vi "Get Clicked Column Header.vi"(0 "TreeControl ref":refnum<vi>, 7 "Coords":T1, 11 "error in (no error)":errorcluster) -> (4 "TreeControl dup ref":refnum<vi>, 8 "Column #":i32, 15 "error out":errorcluster)   [LabVIEW 2015, in "QuickVIew.lvlib"]
doc: "TLB Prime - Application Template 1.3.0.24\nNorm Kirchner, NI Systems Engineering - NI\nCopyright (c) 2014, NI"
uses:
  QuickVIew.lvlib
  <vilib>/Utility/miscctls.llb/LVPoint32TypeDef.ctl
panel:
  # "VI LOCALS"
  # "VI OUTPUTS"
  # "VI INPUTS"
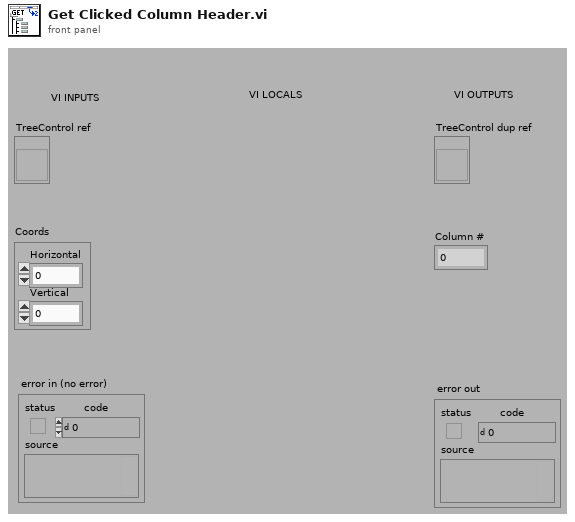
[diagram p1: front panel]
types:
  T1 = typedef "LVPoint32TypeDef.ctl" = cluster{"Horizontal":i32, "Vertical":i32}
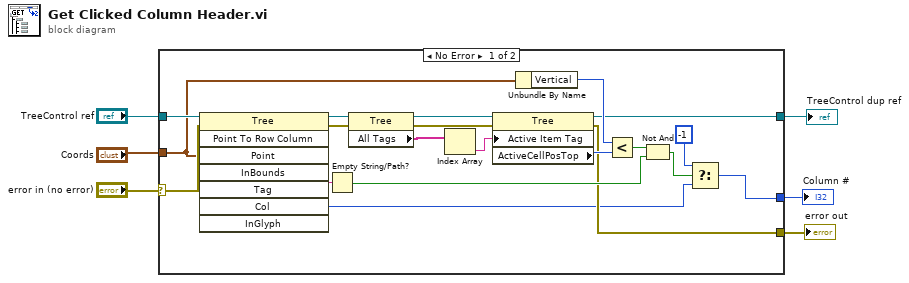
[diagram p0: block diagram]
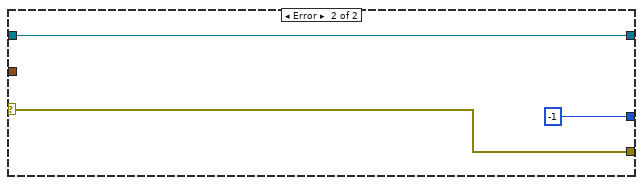
[diagram p2: hidden frame]
diagram:
  n1 = case shown="No Error" "error in (no error)" {
    selector: "error in (no error)" -> [w26 w27]
    tunnel: "TreeControl ref" -> [w25 w28]
    tunnel: "Coords" -> [w22 _]
    tunnel: [w7 -1 ("Col")] -> w4
    tunnel: [w12 w28] -> w2
    tunnel: [w9 w27] -> w1
    frame No Error {
      n2 = invoke on="Invoke Node" class="Tree" method="Point To Row Column"(reference=w25, error in=w26, "Point"=w22) -> (reference out=w23:refnum<vi>, error out=w11:errorcluster, "Tag"=w24:string, "Col"=w8:i32)  [unwired: 5 in, 4 out]
      n3 = Empty String/Path?(string/path=w24) -> (empty?=w15:bool)
      n4 = property class="Tree"(reference=w23, error in=w11) -> (reference out=w21:refnum<vi>, error out=w10:errorcluster, "All Tags"=w20:string[])
      n5 = Index Array(array=w20) -> (element=w19:string)  [unwired: 1 in]
      n6 = property class="Tree"(reference=w21, error in=w10, "Active Item Tag"=w19) -> (reference out=w12:refnum<vi>, error out=w9:errorcluster, "ActiveCellPosTop"=w17:i32)
      n7 = Unbundle By Name(w22) -> ("Vertical"=w18:i32)
      n8 = Less?(x=w18, y=w17) -> (x < y?=w16:bool)
      n9 = Not And(1:w15, 2:w16) -> (0:w14:bool)
      n10 = Select(t=-1 ("Column"), s=w14, f=w8) -> (s? t:f=w7:i32)
    }
    frame Error {
    }
  }
  "Column #" <- w4
  "error out" <- w1
  "TreeControl dup ref" <- w2
